vi "SetDefaults.vi"(8 "error in (no error)":errorcluster, 11 "ArgumentParser in":refnum<class "ArgumentParser.lvclass">) -> (0 "error out":errorcluster, 3 "ArgumentParser out":refnum<class "ArgumentParser.lvclass">)   [LabVIEW 2022 SP3, in "ArgumentParser.lvlib" / "ArgumentParser.lvclass"]
uses:
  ArgumentParser.lvclass
  ArgumentParser.lvclass/ArgumentParser.ctl
  ArgparseWrapper/ArgparseWrapper.lvclass
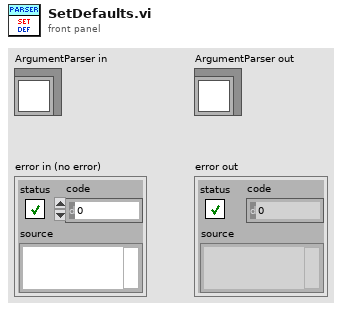
[diagram p1: front panel]
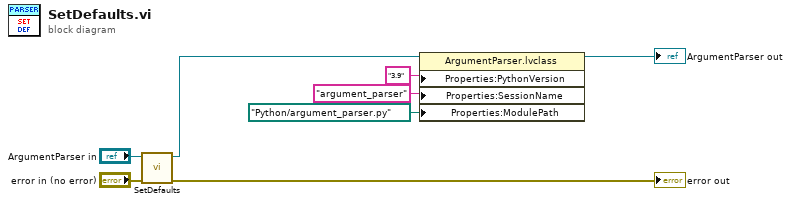
[diagram p0: block diagram]
diagram:
  n1 = call-parent "SetDefaults.vi"("error in (no error)"="error in (no error)", "PythonWrapper in"="ArgumentParser in") -> ("error out"=→"error out":errorcluster, "PythonWrapper out"=w1:refnum<class "ArgumentParser.lvclass">)  [unwired: 8 in]
  n2 = property class="ArgumentParser.lvclass"(reference=w1, "Properties:PythonVersion"="3.9" ("PythonVersion"), "Properties:SessionName"="argument_parser" ("SessionName"), "Properties:ModulePath"=path "Python/argument_parser.py" ("ModulePath")) -> (reference out=→"ArgumentParser out":refnum<class "ArgumentParser.lvclass">)  [unwired: 1 in, 1 out]
